vi "Post-Install Custom Action.vi"(10 "Variant":variant) -> (0 "error out":errorcluster)   [LabVIEW 2011]
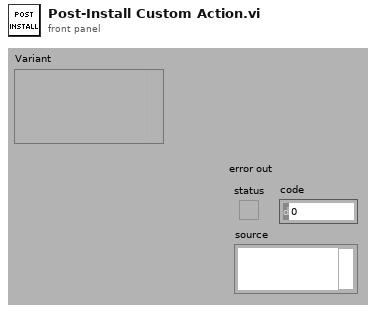
[diagram p1: front panel]
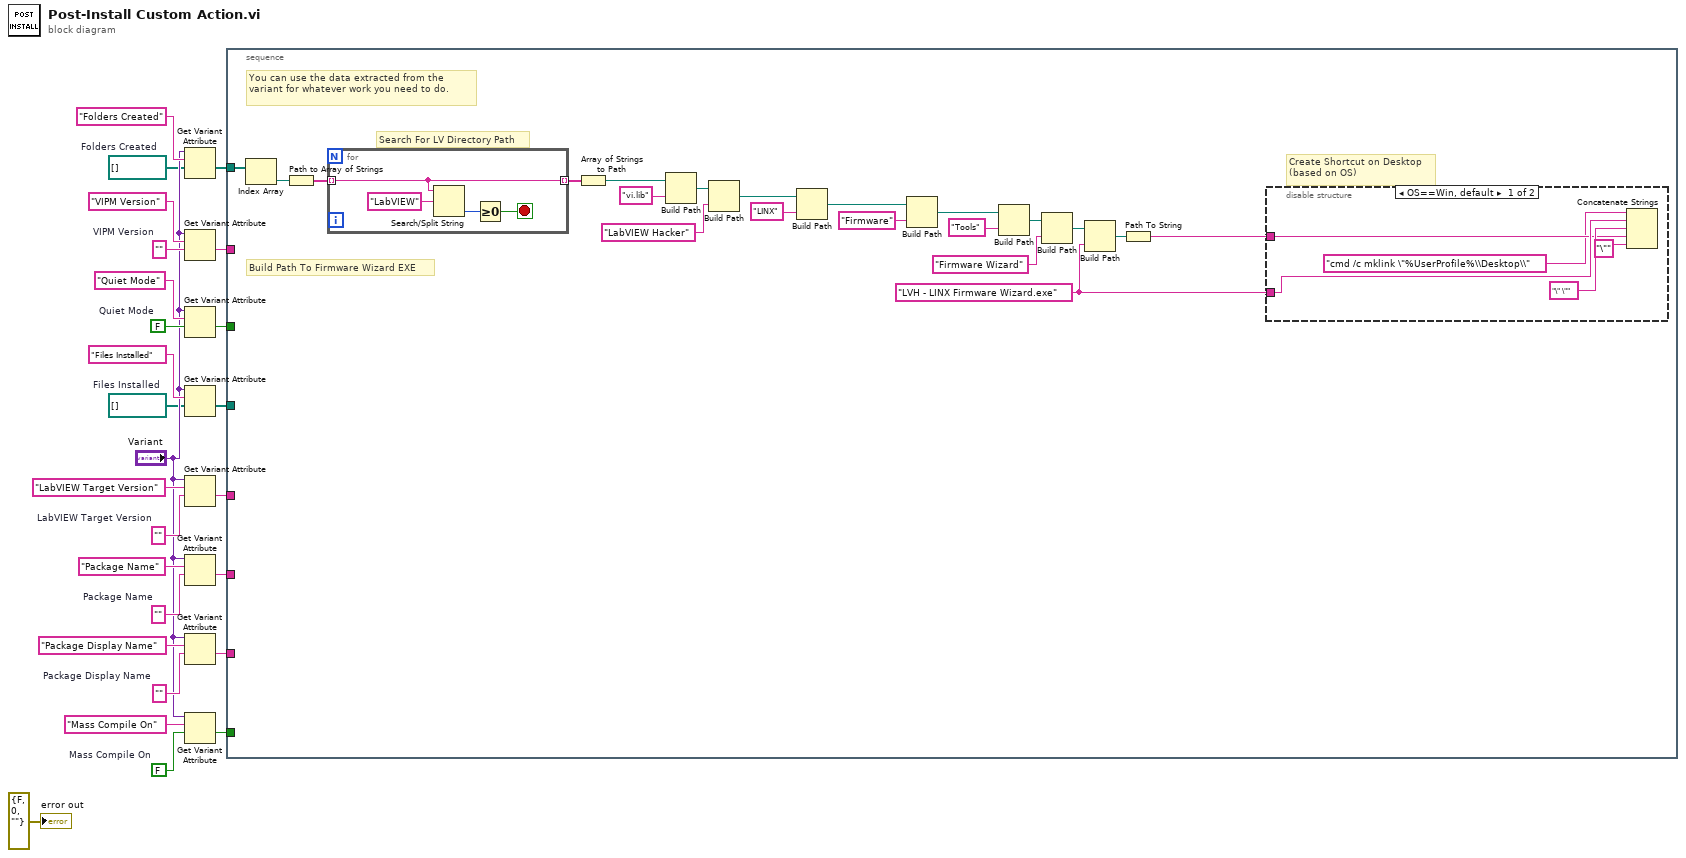
[diagram p0: block diagram]
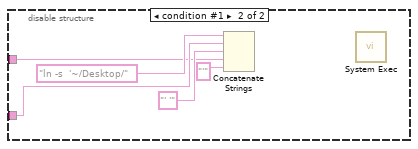
[diagram p2: hidden frame]
diagram:
  w1 = path[] []  # Folders Created
  w2 = path[] []  # Files Installed
  w8 = FALSE  # Mass Compile On
  w9 = ""  # Package Display Name
  w16 = FALSE  # Quiet Mode
  w19 = ""  # VIPM Version
  w21 = ""  # LabVIEW Target Version
  w23 = ""  # Package Name
  n1 = Get Variant Attribute(Variant="Variant", name="Folders Created", default value (empty Variant)=w1) -> (value=w6:path[])  [unwired: 1 in, 3 out]
  n2 = Get Variant Attribute(Variant="Variant", name="VIPM Version", default value (empty Variant)=w19) -> (value=w12:string)  [unwired: 1 in, 3 out]
  n3 = Get Variant Attribute(Variant="Variant", name="Quiet Mode", default value (empty Variant)=w16) -> (value=w11:bool)  [unwired: 1 in, 3 out]
  n4 = Get Variant Attribute(Variant="Variant", name="Files Installed", default value (empty Variant)=w2) -> (value=w5:path[])  [unwired: 1 in, 3 out]
  n5 = Get Variant Attribute(Variant="Variant", name="LabVIEW Target Version", default value (empty Variant)=w21) -> (value=w13:string)  [unwired: 1 in, 3 out]
  n6 = Get Variant Attribute(Variant="Variant", name="Package Name", default value (empty Variant)=w23) -> (value=w14:string)  [unwired: 1 in, 3 out]
  n7 = Get Variant Attribute(Variant="Variant", name="Package Display Name", default value (empty Variant)=w9) -> (value=w15:string)  [unwired: 1 in, 3 out]
  n8 = Get Variant Attribute(Variant="Variant", name="Mass Compile On", default value (empty Variant)=w8) -> (value=w10:bool)  [unwired: 1 in, 3 out]
  n9 = stacked-sequence {
    tunnel: w15 -> [_]
    tunnel: w14 -> [_]
    tunnel: w13 -> [_]
    tunnel: w12 -> [_]
    tunnel: w11 -> [_]
    tunnel: w10 -> [_]
    tunnel: w5 -> [_]
    tunnel: w6 -> [w46]
    frame #0 {
      w29 = "LVH - LINX Firmware Wizard.exe" ("name or relative path")
      # "Create Shortcut on Desktop\n(based on OS)"
      # "Build Path To Firmware Wizard EXE"
      # "Search For LV Directory Path"
      # "You can use the data extracted from the variant for whatever work you need to do."
      n10 = Index Array(array=w46) -> (element=w45:path)  [unwired: 1 in]
      n11 = Path to Array of Strings(0:w45) -> (2:w44:string[])  [unwired: 1 out]
      n12 = for {
        tunnel: w44 -> [w57] mode=indexing
        tunnel: [w57] -> w43 mode=indexing
        stop <- w58 stop-if-true
        n13 = Search/Split String(string=w57, search string/char (-)="LabVIEW") -> (offset of match=w59:i32)  [unwired: 1 in, 2 out]
        n14 = Greater Or Equal To 0?(x=w59) -> (x >= 0?=w58:bool)
      }
      n15 = Array of Strings to Path(0:w43) -> (2:w42:path)  [unwired: 1 in]
      n16 = Build Path(base path=w42, name or relative path="vi.lib") -> (appended path=w39:path)
      n17 = Build Path(base path=w39, name or relative path="LabVIEW Hacker") -> (appended path=w37:path)
      n18 = Build Path(base path=w37, name or relative path="LINX") -> (appended path=w35:path)
      n19 = Build Path(base path=w35, name or relative path="Firmware") -> (appended path=w33:path)
      n20 = Build Path(base path=w33, name or relative path="Tools") -> (appended path=w32:path)
      n21 = Build Path(base path=w32, name or relative path="Firmware Wizard") -> (appended path=w30:path)
      n22 = Build Path(base path=w30, name or relative path=w29) -> (appended path=w28:path)
      n23 = Path To String(path=w28) -> (string=w27:string)
      n24 = disable-structure shown="OS==Win, default" {
        disable-tunnel: w29 -> [w51 w55]
        disable-tunnel: w27 -> [w49 w53]
        frame condition #0 (active) {
          n25 = Concatenate Strings("cmd /c mklink \"%UserProfile%\\Desktop\\", w51, "\" \"" ("string"), w49, "\"" ("string")) -> ()  [unwired: 1 out]
        }
        frame condition #1 {
          n26 = Concatenate Strings("ln -s  '~/Desktop/" ("string"), w55, "' '" ("string"), w53, "'" ("string")) -> ()  [unwired: 1 out]
          n27 = call <vilib>:"System Exec.vi"() -> ()  [unwired: 8 in, 4 out]
        }
      }
    }
  }
  "error out" <- errorcluster {"status"=FALSE, "code"=0, "source"=""} ("error out")
